vi "Init Group.vi"(8 "error in (no error)":errorcluster, 11 "Group BOOL in":refnum<class "Group BOOL.lvclass">) -> (0 "error out":errorcluster, 3 "Group BOOL out":refnum<class "Group BOOL.lvclass">)   [LabVIEW 2020, in "Vecto.lvlib" / "Group BOOL.lvclass"]
uses:
  Group BOOL.lvclass
  Group/Group.lvclass
  Group Config/Group Config.lvclass
  Ref.ctl
  C:/dev/lv20CE/relink/lv-vecto/Vecto/Group/Group.lvclass
  C:/dev/lv20CE/relink/lv-vecto/Vecto/Group BOOL/Group BOOL.lvclass
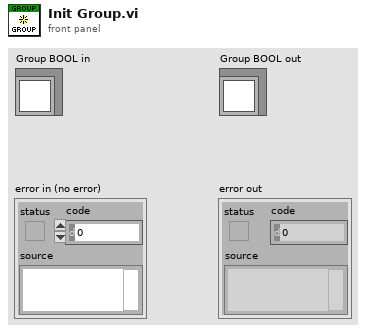
[diagram p1: front panel]
types:
  T1 = typedef "Vecto.lvlib/Group BOOL.lvclass/Ref.ctl" = cluster{"Scaled":bool[], "Timestamp":dbl[], "Raw":bool[]}
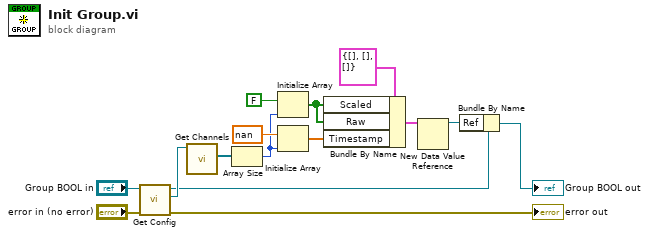
[diagram p0: block diagram]
diagram:
  n1 = call "Get Config.vi"("error in (no error)"="error in (no error)", "Group in"="Group BOOL in") -> ("error out"=→"error out":errorcluster, "Config"=w14:refnum<class "Group Config.lvclass">, "Group out"=w10:refnum<class "Group BOOL.lvclass">)  [unwired: 7 in]
  n2 = call "Get Channels.vi"("Group Config in"=w14) -> ("Channels"=w13:refnum<class "Channel Config.lvclass">[])  [unwired: 8 in, 2 out]
  n3 = Array Size(array=w13) -> (size(s)=w8:i32)
  n4 = Initialize Array(FALSE, w8) -> (w4:bool[])
  n5 = Initialize Array(nan ("element"), w8) -> (w5:dbl[])
  n6 = Bundle By Name(cluster=T1 {"Scaled"=[], "Timestamp"=[], "Raw"=[]} ("Ref"), "Scaled"=w4, "Raw"=w4, "Timestamp"=w5) -> (w3:T1)
  n7 = New Data Value Reference(data value=w3) -> (data value reference=w1:refnum<data-value>)  [unwired: 1 in, 1 out]
  n8 = Bundle By Name(cluster=w10, "Ref"=w1) -> (→"Group BOOL out":refnum<class "Group BOOL.lvclass">)
